vi "sub_rtmain_fgv.vi"(7 "cmd":enum16{"ini", "read", "write", "close"}(ring), 8 "error in":errorcluster, 11 "setpoint":i16) -> (0 "error out":errorcluster, 1 "states":dbl[](array[numeric]), 2 "busy":bool, 3 "off_track":bool)   [LabVIEW 2018]
uses:
  <vilib>/rvi/interface/nirviOpenFPGA/nirviOpenFPGA.xnode
  <vilib>/rvi/interface/nirviCloseFPGA/nirviCloseFPGA.xnode
  <vilib>/rvi/interface/nirviReadWriteControl/nirviReadWriteControl.xnode
  <vilib>/Utility/error.llb/Error Cluster From Error Code.vi
  <vilib>/rvi/interface/Simulation/niFpgaSimulationCallBeginRW.vi
  <vilib>/rvi/errors/niLvFpgaAdjustHostInterfaceError.vi
  <vilib>/addons/control/pid/NI_PID_pid.lvlib
  <vilib>/addons/control/pid/pid.llb/PID (DBL).vi
  NiFpgaLv.dll
  <vilib>/FPGAPlugInAG/Dynamic/niLvFpga_Close_Dynamic.vi
  FPGA Bitfiles/DQNcarpolelvsim_FPGATarget_FPGAsmall2_d4itNFSFwjs.lvbitx
  FPGA_small2.vi
  <vilib>/FPGAPlugInAG/myRIO-1900/niLvFpga_Open_myRIO-1900.vi
  <vilib>/rvi/interface/common/dynamic/niFpgaDynamicAddResources.vi
panel:
  in  "dt (s)":dbl=0.001 format="%.3f"
  in  "output range":cluster{"output high":dbl, "output low":dbl}={"output high"=700.0, "output low"=550.0} {"output low" format="%.2f"; "output high" format="%.2f"}
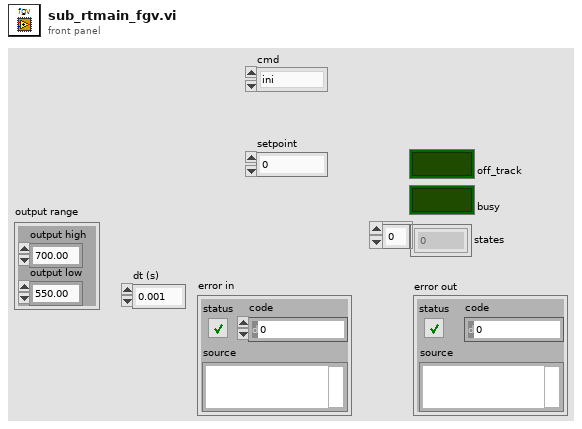
[diagram p1: front panel]
types:
  T1 = cluster{"proportional gain (Kc)":dbl, "integral time (Ti, min)":dbl, "derivative time (Td, min)":dbl}
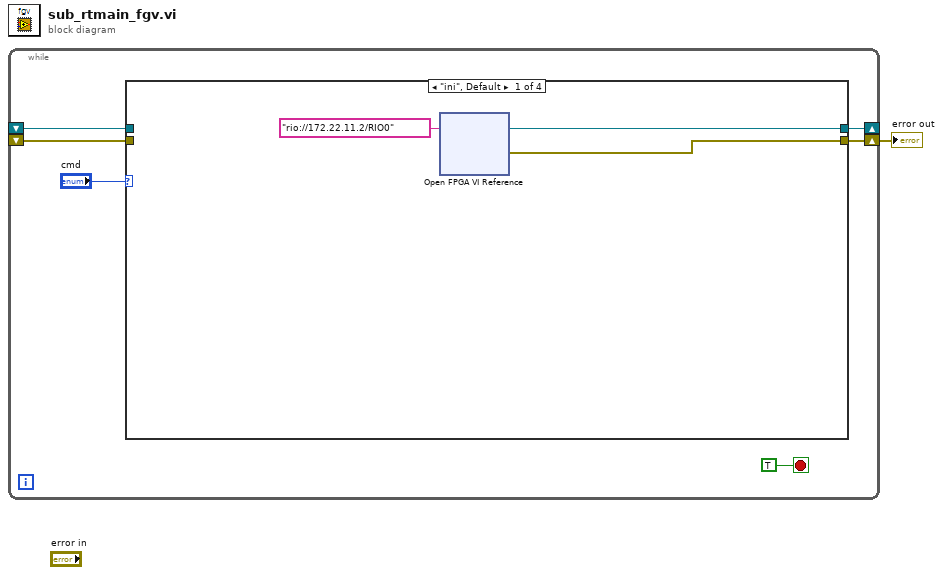
[diagram p0: block diagram]
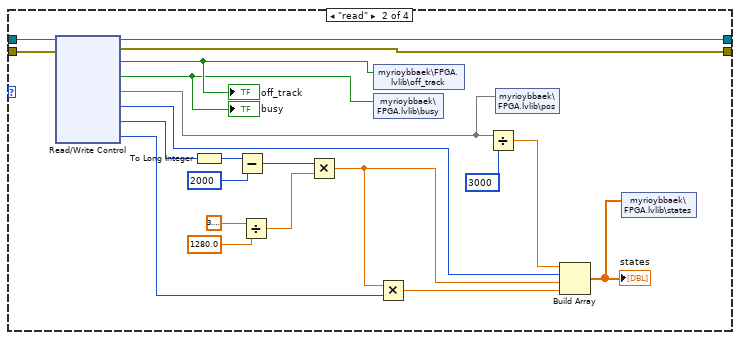
[diagram p2: hidden frame]
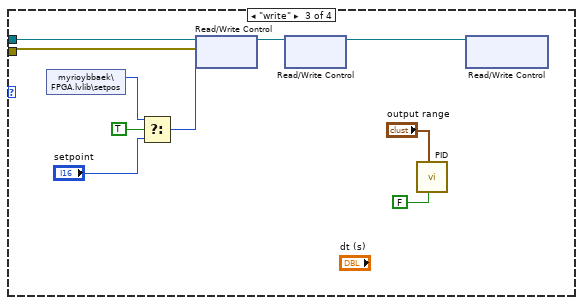
[diagram p3: hidden frame]
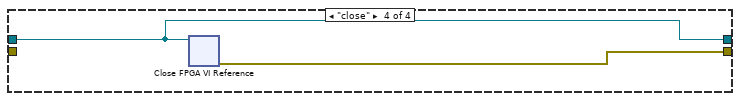
[diagram p4: hidden frame]
diagram:
  n1 = while {
    shift-right: [w5] -> _
    shift-left: _ -> [w4]
    shift-right: [w2] -> w1
    shift-left: _ -> [w3]
    stop <- TRUE stop-if-true
    n2 = case shown="\"ini\", Default" "cmd" {
      tunnel: [w8 w16 _ w45] -> w5
      tunnel: w4 -> [_ w17 w44 w45]
      tunnel: w3 -> [_ w19 w43 _]
      tunnel: [w9 w18 _ w46] -> w2
      frame "ini", Default {
        n3 = xnode "Open FPGA VI Reference"("resource name"=tag "rio://172.22.11.2/RIO0") -> ("FPGA VI Reference Out"=w8:refnum<k20>, "error out"=w9:errorcluster)  [unwired: 1 in]
      }
      frame "read" {
        n4 = xnode "Read/Write Control"("FPGA VI Reference In"=w17, "error in"=w19) -> ("FPGA VI Reference Out"=w16:refnum<k20>, "error out"=w18:errorcluster, "off_track"=w13:bool, "busy"=w12:bool, "pos"=w11, "speed"=w15:i16, "AI0"=w29:u16, "dAI"=w24:i16)
        "off_track" <- w13
        "busy" <- w12
        n5 = To Long Integer(number=w29) -> (32bit integer=w20:i32)
        n6 = Subtract(x=w20, y=u16 2000) -> (x-y=w22:i32)
        n7 = Divide(x=3.141592653589793, y=1280.0) -> (x/y=w21:dbl)
        n8 = Multiply(x=w22, y=w21) -> (x*y=w25:dbl)
        n9 = shared-variable "myrioybbaek\\FPGA.lvlib\\off_track"(w13) -> ()  [unwired: 1 in, 1 out]
        n10 = shared-variable "myrioybbaek\\FPGA.lvlib\\busy"(w12) -> ()  [unwired: 1 in, 1 out]
        n11 = Multiply(x=w25, y=w24) -> (x*y=w23:dbl)
        n12 = Divide(x=w11, y=i16 3000) -> (x/y=w30:dbl)
        n13 = shared-variable "myrioybbaek\\FPGA.lvlib\\pos"(w11) -> ()  [unwired: 1 in, 1 out]
        n14 = Build Array(w30, w15, w25, w23) -> (w14:dbl[])
        "states" <- w14
        n15 = shared-variable "myrioybbaek\\FPGA.lvlib\\states"(w14) -> ()  [unwired: 1 in, 1 out]
      }
      frame "write" {
        n16 = shared-variable "myrioybbaek\\FPGA.lvlib\\setpos"() -> (w41:i16)  [unwired: 1 in, 1 out]
        n17 = Select(t=w41, s=TRUE, f="setpoint") -> (s? t:f=w39:i16)
        n18 = xnode "Read/Write Control"("FPGA VI Reference In"=w44, "error in"=w43, "setpoint"=w39) -> ("FPGA VI Reference Out"=w37:refnum<k20>)  [unwired: 1 out]
        n19 = xnode "Read/Write Control"("FPGA VI Reference In"=w37) -> ("FPGA VI Reference Out"=w38:refnum<k20>)  [unwired: 1 in, 2 out]
        n20 = call-poly <vilib>:"PID.vi"("reinitialize? (F)"=FALSE, "output range"="output range") -> ("dt (s)"=w33:dbl, "PID gains"=w32:T1, "process variable"=w36:dbl)  [unwired: 5 in, 2 out]
        n21 = xnode "Read/Write Control"("FPGA VI Reference In"=w38) -> ()  [unwired: 2 in, 2 out]
      }
      frame "close" {
        n22 = xnode "Close FPGA VI Reference"("FPGA VI Reference In"=w45) -> ("error out"=w46:errorcluster)  [unwired: 1 in]
      }
    }
  }
  "error out" <- w1
